vi "HTUPHTimeToSQLTime.vi"(10 "UPHTime":string) -> (2 "SQL TIME":string)   [LabVIEW 2012]
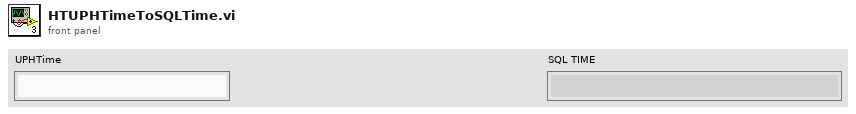
[diagram p1: front panel]
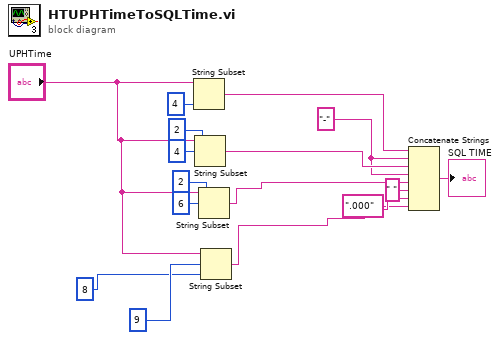
[diagram p0: block diagram]
diagram:
  w7 = "-" ("string")
  n1 = String Subset(string="UPHTime", length (rest)=4 ("length (rest)")) -> (substring=w9:string)  [unwired: 1 in]
  n2 = String Subset(string="UPHTime", offset (0)=4, length (rest)=2 ("length (rest)")) -> (substring=w8:string)
  n3 = String Subset(string="UPHTime", offset (0)=6, length (rest)=2 ("length (rest)")) -> (substring=w6:string)
  n4 = String Subset(string="UPHTime", offset (0)=9, length (rest)=8 ("length (rest)")) -> (substring=w4:string)
  n5 = Concatenate Strings(w9, w7, w8, w7, w6, " " ("string"), w4, ".000" ("string")) -> (→"SQL TIME":string)
